vi "main.vi"() -> ()   [LabVIEW 2016, in "main.lvrbt"]
uses:
  main.lvrbt
  <vilib>/NXT/Subs/MotorOutput.ctl
panel:
  in  "Di":sgl=0.05 format="%#_13g"
  in  "proportional":sgl=0.5 format="%#_13g"
  in  "desired position":i32=320
  in  "Port (All Ports) 2":T1 items=["Port A"=0, "Port B"=1, "Port C"=2, "Ports A & B"=4, "Ports A & C"=5, "Ports B & C"=6, "All Ports"=3]
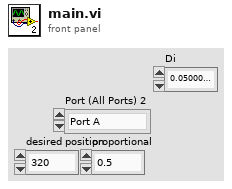
[diagram p1: front panel]
types:
  T1 = typedef "MotorOutput.ctl" = u8
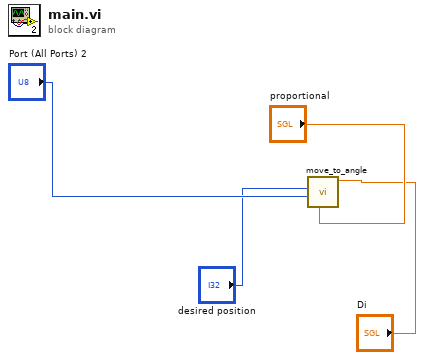
[diagram p0: block diagram]
diagram:
  n1 = call "move_to_angle.vi"("proportional"="proportional", "Port (All Ports)入力"="Port (All Ports) 2", "desired position"="desired position", "Di"="Di") -> ()  [unwired: 8 in]
